vi "Group Check - StateType.vi"(8 "Matched Previous?":bool, 10 "Cross CSM Data (in)":T1={"Name(\"\" to use uuid)"="", "Current State"="", "Arguments"="", "Source Message"={"‘State"="", "’Arguments"="", "’Error"={"status"=FALSE, "code"=0, "source"=""}}, "Source Module"="", "Complete(T)/Start(F)"=FALSE, "LogType"=enum."State Change"}, 11 "GlobalLogFilter.lvclass":refnum<class "LogFilter.lvclass">) -> (0 "Matched? (dup)":bool, 2 "Cross CSM Data":T1={"Name(\"\" to use uuid)"="", "Current State"="", "Arguments"="", "Source Message"={"‘State"="", "’Arguments"="", "’Error"={"status"=FALSE, "code"=0, "source"=""}}, "Source Module"="", "Complete(T)/Start(F)"=FALSE, "LogType"=enum."State Change"}, 3 "GlobalLogFilter.lvclass (dup)":refnum<class "LogFilter.lvclass">)   [LabVIEW 2020, in "Communicable State Machine.lvlib" / "LogFilter.lvclass"]
uses:
  LogFilter.lvclass
  _CSM_GlobalLog_MSG.ctl
  _CSM_Response Source Message.ctl
  _CSM_GlobalLog_MSG_TYPE.ctl
  LogFilter.lvclass/LogFilter.ctl
  Communicable State Machine.lvlib
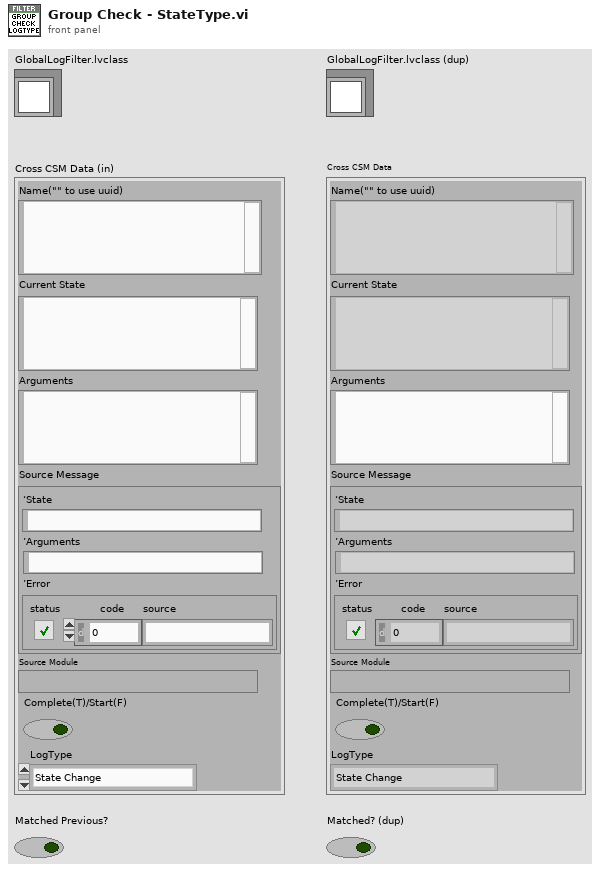
[diagram p1: front panel]
types:
  T1 = typedef "Communicable State Machine.lvlib/_CSM_GlobalLog_MSG.ctl" = cluster{"Name(\"\" to use uuid)":string, "Current State":string, "Arguments":string, "Source Message":T2, "Source Module":string, "Complete(T)/Start(F)":bool, "LogType":T3}
  T2 = typedef "Communicable State Machine.lvlib/_CSM_Response Source Message.ctl" = cluster{"‘State":string, "’Arguments":string, "’Error":errorcluster}
  T3 = typedef "Communicable State Machine.lvlib/_CSM_GlobalLog_MSG_TYPE.ctl" = enum16{"User Log", "State Change", "Status", "Interrupt", "Register", "Unregister", "Error Log", "Module Created", "Module Destroyed"}
  T4 = typedef "Communicable State Machine.lvlib/_CSM_GlobalLog_STATE_TYPE.ctl" = enum16{"State - Internal State", "State - External Message", "State - Response", "State - Complete"}
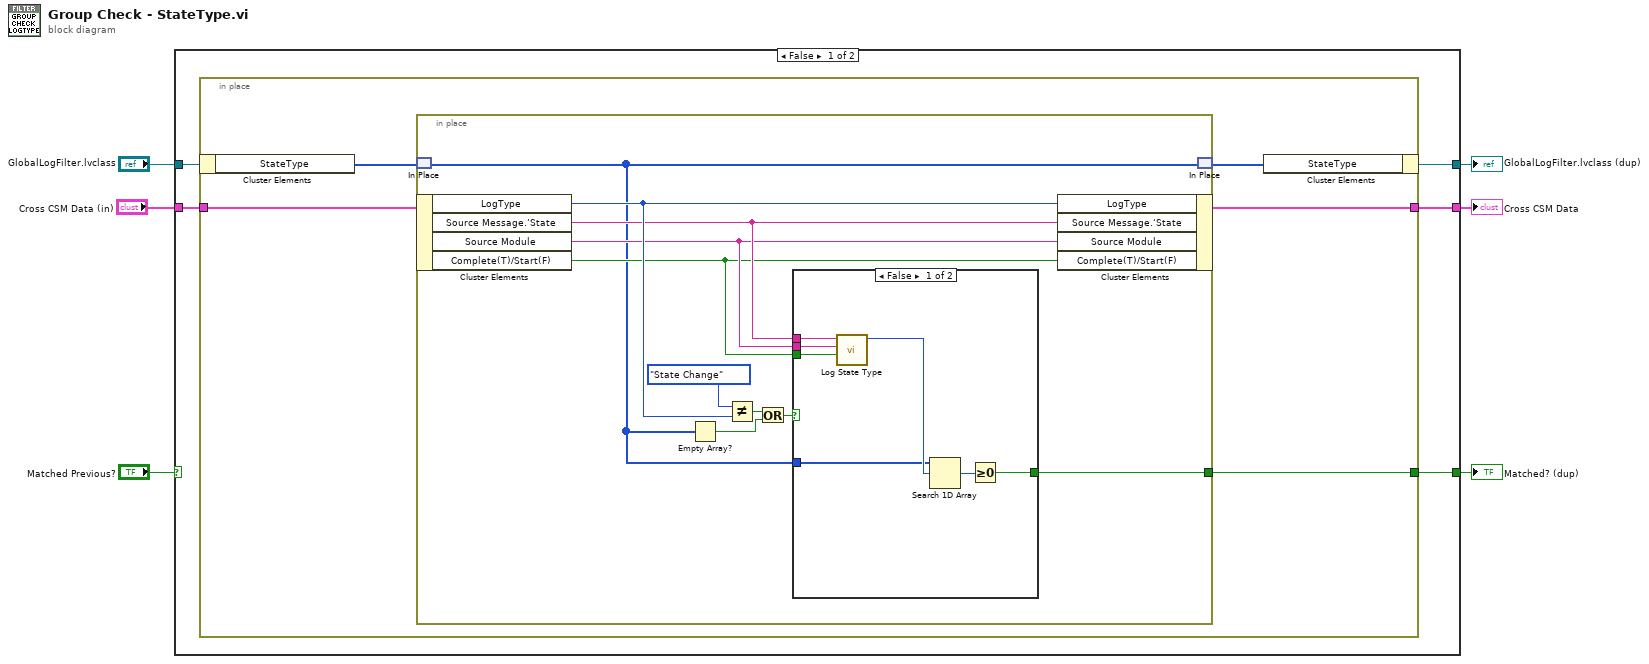
[diagram p0: block diagram]
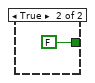
[diagram p2: hidden frame]
diagram:
  n1 = case shown="False" "Matched Previous?" {
    selector: "Matched Previous?" -> [_ w36]
    tunnel: [w10 w37] -> w5
    tunnel: "Cross CSM Data (in)" -> [w11 w37]
    tunnel: [w9 w36] -> w3
    tunnel: [w7 w35] -> w2
    tunnel: "GlobalLogFilter.lvclass" -> [w8 w35]
    frame False {
      n2 = in-place {
        in-place-border: w11 -> [w16]
        in-place-border: [w15] -> w10
        in-place-border: [w14] -> w9
        n3 = in-place-cluster #1(w8) -> ("StateType"=w13:T4[])
        n4 = in-place {
          in-place-border: [w26] -> w14
          n5 = in-place-match #2(w13) -> (w17:T4[])
          n6 = in-place-cluster #3(w16) -> ("LogType"=w25:T3, "Source Message.‘State"=w20:string, "Source Module"=w19:string, "Complete(T)/Start(F)"=w18:bool)
          n7 = Empty Array?(array=w17) -> (empty?=w21:bool)
          n8 = Not Equal?(x=_CSM_GlobalLog_MSG_TYPE."State Change", y=w25) -> (x != y?=w22:bool)
          n9 = Or(x=w22, y=w21) -> (x .or. y?=w23:bool)
          n10 = case shown="False" w23 {
            tunnel: [w29 FALSE] -> w26
            tunnel: w20 -> [w31 _]
            tunnel: w19 -> [w32 _]
            tunnel: w18 -> [w33 _]
            tunnel: w17 -> [w27 _]
            frame False {
              n11 = call "Log State Type.vi"("Complete(T)/Start(F)"=w33, "Source Module"=w32, "‘State"=w31) -> ("CSM_GlobalLog_STATE_TYPE"=w28:T4)  [unwired: 8 in]
              n12 = Search 1D Array(1D array=w27, element=w28) -> (index of element=w30:i32)  [unwired: 1 in]
              n13 = Greater Or Equal To 0?(x=w30) -> (x >= 0?=w29:bool)
            }
            frame True {
            }
          }
          n14 = in-place-cluster #3("LogType"=w25, "Source Message.‘State"=w20, "Source Module"=w19, "Complete(T)/Start(F)"=w18) -> (w15:T1)
          n15 = in-place-match #2(w17) -> (w12:T4[])
        }
        n16 = in-place-cluster #1("StateType"=w12) -> (w7:refnum<class "LogFilter.lvclass">)
      }
    }
    frame True {
    }
  }
  "Cross CSM Data" <- w5
  "Matched? (dup)" <- w3
  "GlobalLogFilter.lvclass (dup)" <- w2
